vi "Test Write Arrays.vi"(11 "TwinCAT ADS in":refnum<class "TwinCAT ADS.lvclass">) -> (3 "TwinCAT ADS out":refnum<class "TwinCAT ADS.lvclass">)   [LabVIEW 2018]
uses:
  TwinCAT ADS Class/TwinCAT ADS.lvclass
  Controls/ST_Complex.ctl
  Controls/Enum.ctl
  Controls/ST_Simple.ctl
  Controls/ST_Packed.ctl
  Controls/FB_Simple.ctl
  257cc43b-7942-4355-97e1-0548d248e4d8.vi
  3c74719b-d65b-41a7-8521-0128952ed356.vi
  cd4f7951-8fa4-40da-833d-fb34ee0c4ef7.vi
  51ef5374-19d2-420c-a3a7-bdd0375b68d3.vi
  a298bf12-7d16-40ed-b77d-c65ab7439937.vi
  05f2186e-a374-4994-a372-07ea411d2204.vi
  23fdef96-acda-4c8c-ba2d-722c4e2ed0c7.vi
  a90a8837-5c87-42c7-8d5a-305d19be2a66.vi
  8e18a9de-928e-4962-8e8c-ac035d36929e.vi
  903064a7-6281-4536-8159-57f8726da337.vi
  TwinCAT ADS Class/VIs/Data/Read.vi
  <vilib>/addons/_JKI Toolkits/Caraya/classes/Assert/Assert Equal Value and Type_Variant.vi
  <vilib>/addons/_JKI Toolkits/Caraya/classes/Assert/Assert True.vi
  <vilib>/addons/_JKI Toolkits/Caraya/classes/Test/Test.lvclass
  <vilib>/addons/_JKI Toolkits/Caraya/classes/Assert/Assert.lvclass
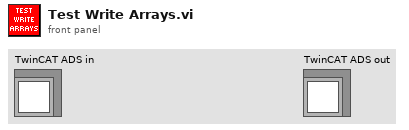
[diagram p1: front panel]
types:
  T1 = typedef "FB_Simple.ctl" = cluster{"_bMember":bool, "_nMember":i32, "_sMember":string}
  T2 = typedef "ST_Complex.ctl" = cluster{"bMember":bool, "eMember":T3, "stSimpleMember":T4, "stPackedMember":T5, "FB_Simple":T1, "arrfMember":dbl[]}
  T3 = typedef "Enum.ctl" = enum16{"Member 0", "Member 1", "Member 2"}
  T4 = typedef "ST_Simple.ctl" = cluster{"bMember":bool, "dtMember":timestamp, "nMember":i32}
  T5 = typedef "ST_Packed.ctl" = cluster{"bMember":bool, "dtMember":timestamp, "fMember":dbl}
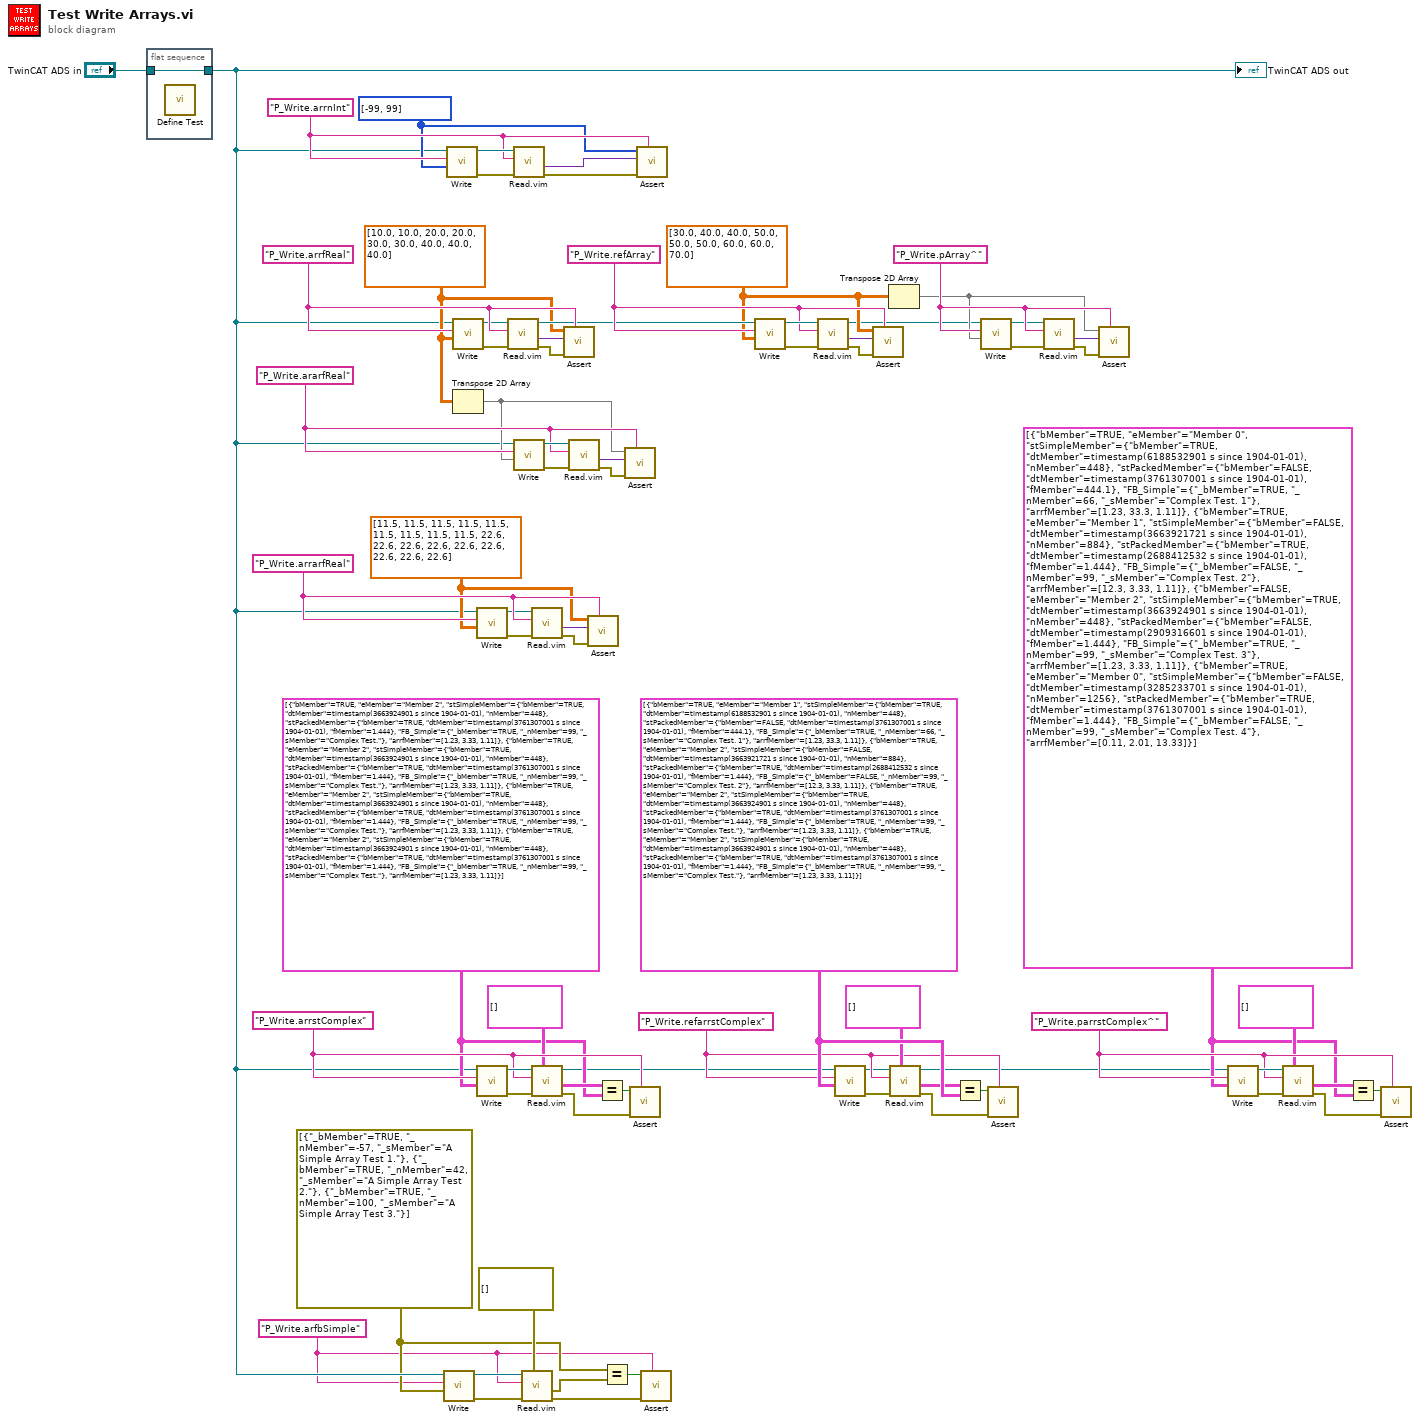
[diagram p0: block diagram]
diagram:
  w2 = "P_Write.arfbSimple" ("Symbol Name")
  w3 = T1[] [{"_bMember"=TRUE, "_nMember"=-57, "_sMember"="A Simple Array Test 1."}, {"_bMember"=TRUE, "_nMember"=42, "_sMember"="A Simple Array Test 2."}, {"_bMember"=TRUE, "_nMember"=100, "_sMember"="A Simple Array Test 3."}]
  w11 = T2[][] [[{"bMember"=TRUE, "eMember"=enum."Member 0", "stSimpleMember"={"bMember"=TRUE, "dtMember"=timestamp(6188532901 s since 1904-01-01), "nMember"=448}, "stPackedMember"={"bMember"=FALSE, "dtMember"=timestamp(3761307001 s since 1904-01-01), "fMember"=444.1}, "FB_Simple"={"_bMember"=TRUE, "_nMember"=66, "_sMember"="Complex Test. 1"}, "arrfMember"=[1.23, 33.3, 1.11]}, {"bMember"=TRUE, "eMember"=enum."Member 1", "stSimpleMember"={"bMember"=FALSE, "dtMember"=timestamp(3663921721 s since 1904-01-01), "nMember"=884}, "stPackedMember"={"bMember"=TRUE, "dtMember"=timestamp(2688412532 s since 1904-01-01), "fMember"=1.444}, "FB_Simple"={"_bMember"=FALSE, "_nMember"=99, "_sMember"="Complex Test. 2"}, "arrfMember"=[12.3, 3.33, 1.11]}], [{"bMember"=FALSE, "eMember"=enum."Member 2", "stSimpleMember"={"bMember"=TRUE, "dtMember"=timestamp(3663924901 s since 1904-01-01), "nMember"=448}, "stPackedMember"={"bMember"=FALSE, "dtMember"=timestamp(2909316601 s since 1904-01-01), "fMember"=1.444}, "FB_Simple"={"_bMember"=TRUE, "_nMember"=99, "_sMember"="Complex Test. 3"}, "arrfMember"=[1.23, 3.33, 1.11]}, {"bMember"=TRUE, "eMember"=enum."Member 0", "stSimpleMember"={"bMember"=FALSE, "dtMember"=timestamp(3285233701 s since 1904-01-01), "nMember"=1256}, "stPackedMember"={"bMember"=TRUE, "dtMember"=timestamp(3761307001 s since 1904-01-01), "fMember"=1.444}, "FB_Simple"={"_bMember"=FALSE, "_nMember"=99, "_sMember"="Complex Test. 4"}, "arrfMember"=[0.11, 2.01, 13.33]}]]
  w15 = "P_Write.parrstComplex^" ("Symbol Name")
  w27 = T2[][] [[{"bMember"=TRUE, "eMember"=enum."Member 1", "stSimpleMember"={"bMember"=TRUE, "dtMember"=timestamp(6188532901 s since 1904-01-01), "nMember"=448}, "stPackedMember"={"bMember"=FALSE, "dtMember"=timestamp(3761307001 s since 1904-01-01), "fMember"=444.1}, "FB_Simple"={"_bMember"=TRUE, "_nMember"=66, "_sMember"="Complex Test. 1"}, "arrfMember"=[1.23, 33.3, 1.11]}, {"bMember"=TRUE, "eMember"=enum."Member 2", "stSimpleMember"={"bMember"=FALSE, "dtMember"=timestamp(3663921721 s since 1904-01-01), "nMember"=884}, "stPackedMember"={"bMember"=TRUE, "dtMember"=timestamp(2688412532 s since 1904-01-01), "fMember"=1.444}, "FB_Simple"={"_bMember"=FALSE, "_nMember"=99, "_sMember"="Complex Test. 2"}, "arrfMember"=[12.3, 3.33, 1.11]}], [{"bMember"=TRUE, "eMember"=enum."Member 2", "stSimpleMember"={"bMember"=TRUE, "dtMember"=timestamp(3663924901 s since 1904-01-01), "nMember"=448}, "stPackedMember"={"bMember"=TRUE, "dtMember"=timestamp(3761307001 s since 1904-01-01), "fMember"=1.444}, "FB_Simple"={"_bMember"=TRUE, "_nMember"=99, "_sMember"="Complex Test."}, "arrfMember"=[1.23, 3.33, 1.11]}, {"bMember"=TRUE, "eMember"=enum."Member 2", "stSimpleMember"={"bMember"=TRUE, "dtMember"=timestamp(3663924901 s since 1904-01-01), "nMember"=448}, "stPackedMember"={"bMember"=TRUE, "dtMember"=timestamp(3761307001 s since 1904-01-01), "fMember"=1.444}, "FB_Simple"={"_bMember"=TRUE, "_nMember"=99, "_sMember"="Complex Test."}, "arrfMember"=[1.23, 3.33, 1.11]}]]
  w23 = "P_Write.refarrstComplex" ("Symbol Name")
  w28 = T2[][] [[{"bMember"=TRUE, "eMember"=enum."Member 2", "stSimpleMember"={"bMember"=TRUE, "dtMember"=timestamp(3663924901 s since 1904-01-01), "nMember"=448}, "stPackedMember"={"bMember"=TRUE, "dtMember"=timestamp(3761307001 s since 1904-01-01), "fMember"=1.444}, "FB_Simple"={"_bMember"=TRUE, "_nMember"=99, "_sMember"="Complex Test."}, "arrfMember"=[1.23, 3.33, 1.11]}, {"bMember"=TRUE, "eMember"=enum."Member 2", "stSimpleMember"={"bMember"=TRUE, "dtMember"=timestamp(3663924901 s since 1904-01-01), "nMember"=448}, "stPackedMember"={"bMember"=TRUE, "dtMember"=timestamp(3761307001 s since 1904-01-01), "fMember"=1.444}, "FB_Simple"={"_bMember"=TRUE, "_nMember"=99, "_sMember"="Complex Test."}, "arrfMember"=[1.23, 3.33, 1.11]}], [{"bMember"=TRUE, "eMember"=enum."Member 2", "stSimpleMember"={"bMember"=TRUE, "dtMember"=timestamp(3663924901 s since 1904-01-01), "nMember"=448}, "stPackedMember"={"bMember"=TRUE, "dtMember"=timestamp(3761307001 s since 1904-01-01), "fMember"=1.444}, "FB_Simple"={"_bMember"=TRUE, "_nMember"=99, "_sMember"="Complex Test."}, "arrfMember"=[1.23, 3.33, 1.11]}, {"bMember"=TRUE, "eMember"=enum."Member 2", "stSimpleMember"={"bMember"=TRUE, "dtMember"=timestamp(3663924901 s since 1904-01-01), "nMember"=448}, "stPackedMember"={"bMember"=TRUE, "dtMember"=timestamp(3761307001 s since 1904-01-01), "fMember"=1.444}, "FB_Simple"={"_bMember"=TRUE, "_nMember"=99, "_sMember"="Complex Test."}, "arrfMember"=[1.23, 3.33, 1.11]}]]
  w32 = "P_Write.arrstComplex" ("Symbol Name")
  w36 = dbl[][][] [[[11.5, 11.5, 11.5], [11.5, 11.5, 11.5], [11.5, 11.5, 11.5]], [[22.6, 22.6, 22.6], [22.6, 22.6, 22.6], [22.6, 22.6, 22.6]]]
  w41 = "P_Write.arrarfReal" ("Symbol Name")
  w44 = "P_Write.ararfReal" ("Symbol Name")
  w56 = "P_Write.pArray^" ("Symbol Name")
  w51 = sgl[][] [[30.0, 40.0, 40.0], [50.0, 50.0, 50.0], [60.0, 60.0, 70.0]]
  w58 = "P_Write.refArray" ("Symbol Name")
  w43 = sgl[][] [[10.0, 10.0, 20.0], [20.0, 30.0, 30.0], [40.0, 40.0, 40.0]]
  w67 = "P_Write.arrfReal" ("Symbol Name")
  w69 = i16[] [-99, 99]
  w70 = "P_Write.arrnInt" ("Symbol Name")
  n1 = flat-sequence {
    tunnel: "TwinCAT ADS in" -> [w75]
    tunnel: [w75] -> w6
    frame #0 {
      n2 = call <vilib>:"Define Test.vi"() -> ()  [unwired: 10 in, 2 out]
    }
  }
  n3 = call "Write.vi"("Value"=w3, "Symbol Name"=w2, "TwinCAT ADS in"=w6) -> ("error out"=w9:errorcluster, "TwinCAT ADS out"=w8:refnum<class "TwinCAT ADS.lvclass">)  [unwired: 7 in]
  n4 = call "Write.vi"("Value"=w69, "Symbol Name"=w70, "TwinCAT ADS in"=w6) -> ("error out"=w72:errorcluster, "TwinCAT ADS out"=w73:refnum<class "TwinCAT ADS.lvclass">)  [unwired: 7 in]
  n5 = call "Write.vi"("Value"=w43, "Symbol Name"=w67, "TwinCAT ADS in"=w6) -> ("error out"=w65:errorcluster, "TwinCAT ADS out"=w64:refnum<class "TwinCAT ADS.lvclass">)  [unwired: 7 in]
  n6 = Transpose 2D Array(2D array=w43) -> (transposed array=w42:sgl[][])
  n7 = call "Write.vi"("Value"=w36, "Symbol Name"=w41, "TwinCAT ADS in"=w6) -> ("error out"=w39:errorcluster, "TwinCAT ADS out"=w38:refnum<class "TwinCAT ADS.lvclass">)  [unwired: 7 in]
  n8 = call "Write.vi"("Value"=w28, "Symbol Name"=w32, "TwinCAT ADS in"=w6) -> ("error out"=w34:errorcluster, "TwinCAT ADS out"=w35:refnum<class "TwinCAT ADS.lvclass">)  [unwired: 7 in]
  n9 = call "Read.vim"("error in (no error)"=w65, "Symbol Name"=w67, "TwinCAT ADS in"=w64) -> ("error out"=w66:errorcluster, "Value"=w63:variant, "TwinCAT ADS out"=w57:refnum<class "TwinCAT ADS.lvclass">)  [unwired: 6 in]
  n10 = call "Read.vim"("error in (no error)"=w72, "Symbol Name"=w70, "TwinCAT ADS in"=w73) -> ("error out"=w71:errorcluster, "Value"=w68:variant)  [unwired: 6 in, 1 out]
  n11 = call "Write.vi"("Value"=w42, "Symbol Name"=w44, "TwinCAT ADS in"=w6) -> ("error out"=w46:errorcluster, "TwinCAT ADS out"=w47:refnum<class "TwinCAT ADS.lvclass">)  [unwired: 7 in]
  n12 = call "Read.vim"("Type"=T1[] [], "error in (no error)"=w9, "Symbol Name"=w2, "TwinCAT ADS in"=w8) -> ("error out"=w1:errorcluster, "Value"=w4:T1[])  [unwired: 5 in, 1 out]
  n13 = call "Read.vim"("error in (no error)"=w39, "Symbol Name"=w41, "TwinCAT ADS in"=w38) -> ("error out"=w40:errorcluster, "Value"=w37:variant)  [unwired: 6 in, 1 out]
  n14 = call "Read.vim"("Type"=T2[][] [], "error in (no error)"=w34, "Symbol Name"=w32, "TwinCAT ADS in"=w35) -> ("error out"=w33:errorcluster, "Value"=w30:T2[][], "TwinCAT ADS out"=w19:refnum<class "TwinCAT ADS.lvclass">)  [unwired: 5 in]
  n15 = call-poly <vilib>:"Assert.vi"("Label"=w67, "error in (no error)"=w66, "Y"=w63, "X"=w43) -> ()  [unwired: 6 in, 2 out]
  n16 = call "Read.vim"("error in (no error)"=w46, "Symbol Name"=w44, "TwinCAT ADS in"=w47) -> ("error out"=w45:errorcluster, "Value"=w48:variant)  [unwired: 6 in, 1 out]
  n17 = call-poly <vilib>:"Assert.vi"("Label"=w41, "error in (no error)"=w40, "Y"=w37, "X"=w36) -> ()  [unwired: 6 in, 2 out]
  n18 = Equal?(x=w30, y=w28) -> (x = y?=w29:bool)
  n19 = Equal?(x=w3, y=w4) -> (x = y?=w5:bool)
  n20 = call-poly <vilib>:"Assert.vi"("Label"=w44, "error in (no error)"=w45, "Y"=w48, "X"=w42) -> ()  [unwired: 6 in, 2 out]
  n21 = call-poly <vilib>:"Assert.vi"("Label"=w32, "error in (no error)"=w33, "True?"=w29) -> ()  [unwired: 7 in, 2 out]
  n22 = call-poly <vilib>:"Assert.vi"("Label"=w70, "error in (no error)"=w71, "Y"=w68, "X"=w69) -> ()  [unwired: 6 in, 2 out]
  n23 = call-poly <vilib>:"Assert.vi"("Label"=w2, "error in (no error)"=w1, "True?"=w5) -> ()  [unwired: 7 in, 2 out]
  n24 = call "Write.vi"("Value"=w51, "Symbol Name"=w58, "TwinCAT ADS in"=w57) -> ("error out"=w60:errorcluster, "TwinCAT ADS out"=w61:refnum<class "TwinCAT ADS.lvclass">)  [unwired: 7 in]
  n25 = call "Read.vim"("error in (no error)"=w60, "Symbol Name"=w58, "TwinCAT ADS in"=w61) -> ("error out"=w59:errorcluster, "Value"=w62:variant, "TwinCAT ADS out"=w49:refnum<class "TwinCAT ADS.lvclass">)  [unwired: 6 in]
  n26 = call "Write.vi"("Value"=w27, "Symbol Name"=w23, "TwinCAT ADS in"=w19) -> ("error out"=w21:errorcluster, "TwinCAT ADS out"=w20:refnum<class "TwinCAT ADS.lvclass">)  [unwired: 7 in]
  n27 = call-poly <vilib>:"Assert.vi"("Label"=w58, "error in (no error)"=w59, "Y"=w62, "X"=w51) -> ()  [unwired: 6 in, 2 out]
  n28 = Transpose 2D Array(2D array=w51) -> (transposed array=w50:sgl[][])
  n29 = call "Read.vim"("Type"=T2[][] [], "error in (no error)"=w21, "Symbol Name"=w23, "TwinCAT ADS in"=w20) -> ("error out"=w22:errorcluster, "Value"=w25:T2[][], "TwinCAT ADS out"=w10:refnum<class "TwinCAT ADS.lvclass">)  [unwired: 5 in]
  n30 = Equal?(x=w25, y=w27) -> (x = y?=w26:bool)
  n31 = call "Write.vi"("Value"=w50, "Symbol Name"=w56, "TwinCAT ADS in"=w49) -> ("error out"=w54:errorcluster, "TwinCAT ADS out"=w53:refnum<class "TwinCAT ADS.lvclass">)  [unwired: 7 in]
  n32 = call-poly <vilib>:"Assert.vi"("Label"=w23, "error in (no error)"=w22, "True?"=w26) -> ()  [unwired: 7 in, 2 out]
  n33 = call "Read.vim"("error in (no error)"=w54, "Symbol Name"=w56, "TwinCAT ADS in"=w53) -> ("error out"=w55:errorcluster, "Value"=w52:variant)  [unwired: 6 in, 1 out]
  n34 = call-poly <vilib>:"Assert.vi"("Label"=w56, "error in (no error)"=w55, "Y"=w52, "X"=w50) -> ()  [unwired: 6 in, 2 out]
  n35 = call "Write.vi"("Value"=w11, "Symbol Name"=w15, "TwinCAT ADS in"=w10) -> ("error out"=w17:errorcluster, "TwinCAT ADS out"=w18:refnum<class "TwinCAT ADS.lvclass">)  [unwired: 7 in]
  n36 = call "Read.vim"("Type"=T2[][] [], "error in (no error)"=w17, "Symbol Name"=w15, "TwinCAT ADS in"=w18) -> ("error out"=w16:errorcluster, "Value"=w13:T2[][])  [unwired: 5 in, 1 out]
  n37 = Equal?(x=w13, y=w11) -> (x = y?=w12:bool)
  n38 = call-poly <vilib>:"Assert.vi"("Label"=w15, "error in (no error)"=w16, "True?"=w12) -> ()  [unwired: 7 in, 2 out]
  "TwinCAT ADS out" <- w6
